vi "TriggeredHistogram10.vi"(7 "Last laser in":bool, 9 "Histogram in":u16[](array[numeric])=[0, 0, 0, 0, 0, 0, 0, 0, 0, 0], 10 "PMT 20bit in":bool[](array[boolean])=[FALSE, FALSE, FALSE, FALSE, FALSE, FALSE, FALSE, FALSE, FALSE, FALSE, FALSE, FALSE, FALSE, FALSE, FALSE, FALSE, FALSE, FALSE, FALSE, FALSE], 11 "Laser 10bit in":bool[](array[boolean])=[FALSE, FALSE, FALSE, FALSE, FALSE, FALSE, FALSE, FALSE, FALSE, FALSE]) -> (1 "Histogram out":u16[](array[numeric]))   [LabVIEW 2012]
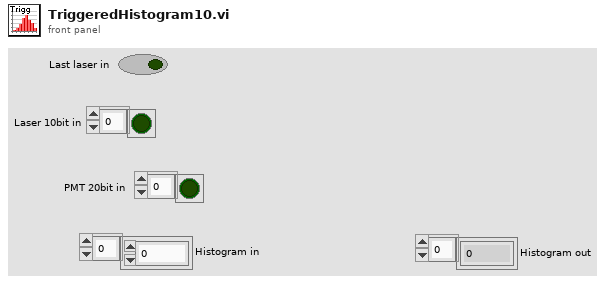
[diagram p1: front panel]
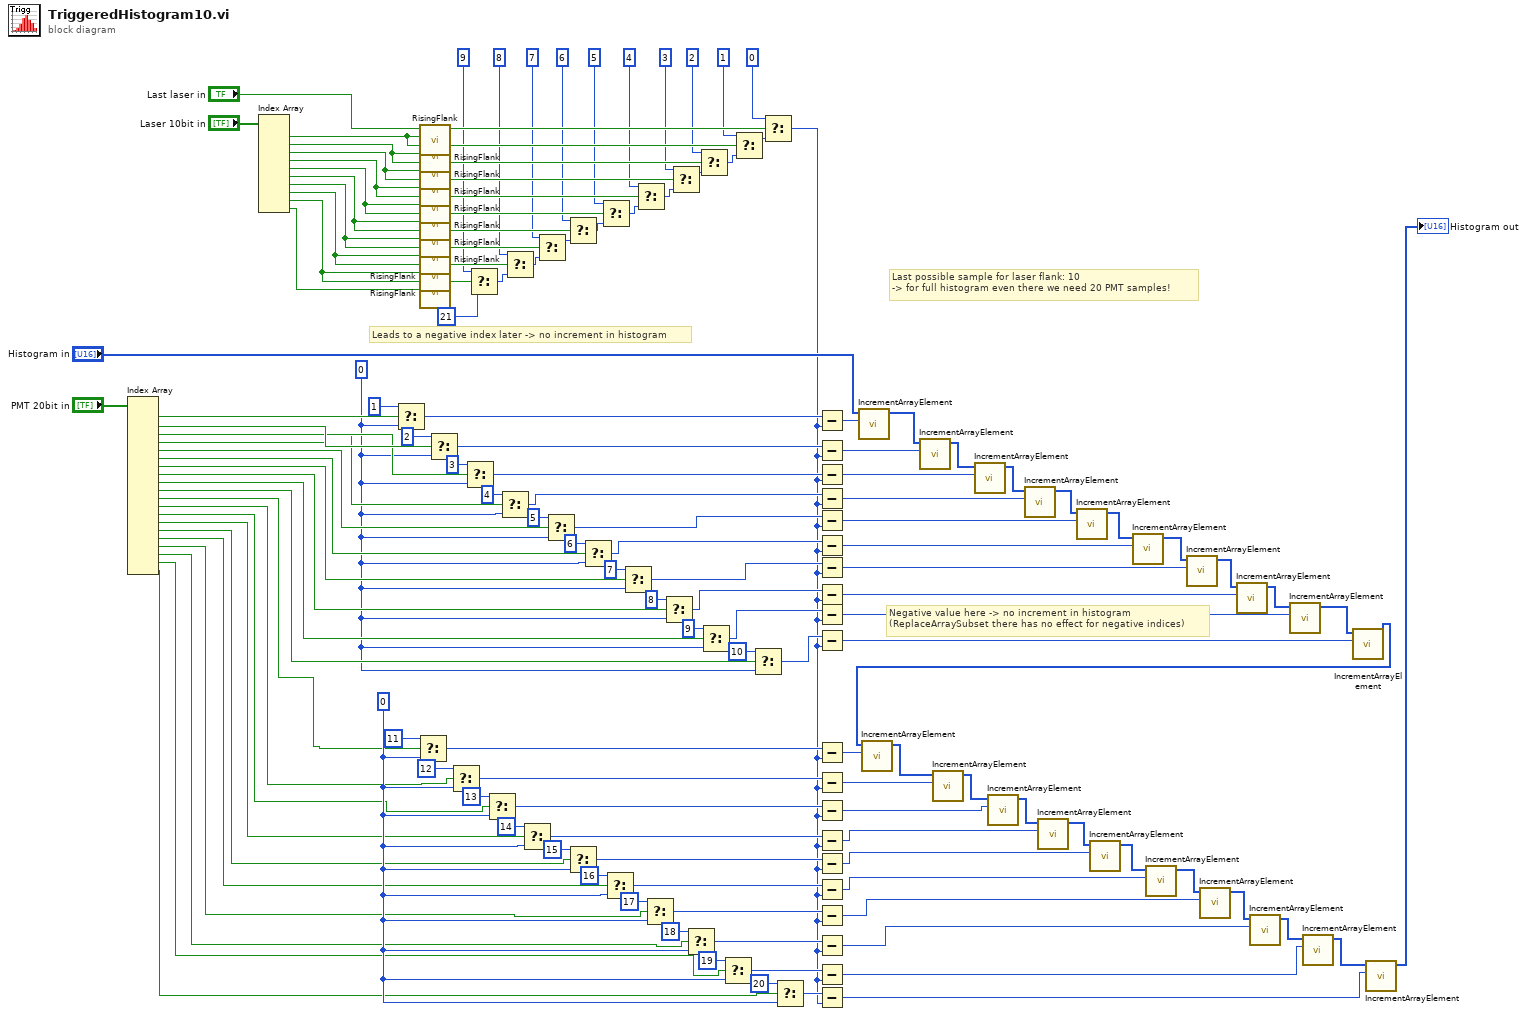
[diagram p0: block diagram]
diagram:
  w43 = 0 ("f")
  w84 = 0 ("f")
  # "Last possible sample for laser flank: 10\n-> for full histogram even there we need 20 PMT samples!"
  # "Leads to a negative index later -> no increment in histogram"
  # "Negative value here -> no increment in histogram\n(ReplaceArraySubset there has no effect for negative indices)"
  n1 = Index Array(array="PMT 20bit in") -> (element #1=w104:bool, element #2=w102:bool, element #3=w100:bool, element #4=w97:bool, element #5=w95:bool, element #6=w93:bool, element #7=w91:bool, element #8=w89:bool, element #9=w87:bool, element #10=w85:bool, element #11=w42:bool, element #12=w41:bool, element #13=w40:bool, element #14=w39:bool, element #15=w38:bool, element #16=w37:bool, element #17=w36:bool, element #18=w35:bool, element #19=w34:bool, element #20=w33:bool)  [unwired: 20 in]
  n2 = Index Array(array="Laser 10bit in") -> (element #1=w146:bool, element #2=w145:bool, element #3=w144:bool, element #4=w143:bool, element #5=w142:bool, element #6=w141:bool, element #7=w140:bool, element #8=w139:bool, element #9=w138:bool, element #10=w137:bool)  [unwired: 10 in]
  n3 = Select(t=1, s=w104, f=w84) -> (s? t:f=w83:i32)
  n4 = Select(t=11, s=w42, f=w43) -> (s? t:f=w32:i32)
  n5 = call "RisingFlank.vi"("2nd sample"=w146, "1st sample"="Last laser in") -> ("Rising flank?"=w136:bool)  [unwired: 7 in]
  n6 = call "RisingFlank.vi"("2nd sample"=w145, "1st sample"=w146) -> ("Rising flank?"=w133:bool)  [unwired: 7 in]
  n7 = call "RisingFlank.vi"("2nd sample"=w144, "1st sample"=w145) -> ("Rising flank?"=w132:bool)  [unwired: 7 in]
  n8 = call "RisingFlank.vi"("2nd sample"=w143, "1st sample"=w144) -> ("Rising flank?"=w131:bool)  [unwired: 7 in]
  n9 = call "RisingFlank.vi"("2nd sample"=w142, "1st sample"=w143) -> ("Rising flank?"=w130:bool)  [unwired: 7 in]
  n10 = call "RisingFlank.vi"("2nd sample"=w141, "1st sample"=w142) -> ("Rising flank?"=w129:bool)  [unwired: 7 in]
  n11 = call "RisingFlank.vi"("2nd sample"=w140, "1st sample"=w141) -> ("Rising flank?"=w128:bool)  [unwired: 7 in]
  n12 = call "RisingFlank.vi"("2nd sample"=w139, "1st sample"=w140) -> ("Rising flank?"=w127:bool)  [unwired: 7 in]
  n13 = call "RisingFlank.vi"("2nd sample"=w138, "1st sample"=w139) -> ("Rising flank?"=w126:bool)  [unwired: 7 in]
  n14 = call "RisingFlank.vi"("2nd sample"=w137, "1st sample"=w138) -> ("Rising flank?"=w125:bool)  [unwired: 7 in]
  n15 = Select(t=2, s=w102, f=w84) -> (s? t:f=w82:i32)
  n16 = Select(t=12, s=w41, f=w43) -> (s? t:f=w31:i32)
  n17 = Select(t=3, s=w100, f=w84) -> (s? t:f=w77:i32)
  n18 = Select(t=9 ("Insert index"), s=w125, f=21) -> (s? t:f=w109:i32)
  n19 = Select(t=13, s=w40, f=w43) -> (s? t:f=w30:i32)
  n20 = Select(t=4, s=w97, f=w84) -> (s? t:f=w76:i32)
  n21 = Select(t=8 ("Insert index"), s=w126, f=w109) -> (s? t:f=w111:i32)
  n22 = Select(t=14, s=w39, f=w43) -> (s? t:f=w29:i32)
  n23 = Select(t=7 ("Insert index"), s=w127, f=w111) -> (s? t:f=w113:i32)
  n24 = Select(t=5, s=w95, f=w84) -> (s? t:f=w75:i32)
  n25 = Select(t=6 ("Insert index"), s=w128, f=w113) -> (s? t:f=w115:i32)
  n26 = Select(t=15, s=w38, f=w43) -> (s? t:f=w28:i32)
  n27 = Select(t=6, s=w93, f=w84) -> (s? t:f=w74:i32)
  n28 = Select(t=5 ("Insert index"), s=w129, f=w115) -> (s? t:f=w117:i32)
  n29 = Select(t=16, s=w37, f=w43) -> (s? t:f=w27:i32)
  n30 = Select(t=7, s=w91, f=w84) -> (s? t:f=w73:i32)
  n31 = Select(t=4 ("Insert index"), s=w130, f=w117) -> (s? t:f=w119:i32)
  n32 = Select(t=17, s=w36, f=w43) -> (s? t:f=w26:i32)
  n33 = Select(t=8, s=w89, f=w84) -> (s? t:f=w72:i32)
  n34 = Select(t=3 ("Insert index"), s=w131, f=w119) -> (s? t:f=w122:i32)
  n35 = Select(t=18, s=w35, f=w43) -> (s? t:f=w25:i32)
  n36 = Select(t=2 ("Insert index"), s=w132, f=w122) -> (s? t:f=w124:i32)
  n37 = Select(t=9, s=w87, f=w84) -> (s? t:f=w71:i32)
  n38 = Select(t=19, s=w34, f=w43) -> (s? t:f=w24:i32)
  n39 = Select(t=1 ("Insert index"), s=w133, f=w124) -> (s? t:f=w134:i32)
  n40 = Select(t=10, s=w85, f=w84) -> (s? t:f=w70:i32)
  n41 = Select(t=0 ("Insert index"), s=w136, f=w134) -> (s? t:f=w22:i32)
  n42 = Select(t=20, s=w33, f=w43) -> (s? t:f=w23:i32)
  n43 = Subtract(x=w83, y=w22) -> (x-y=w80:i32)
  n44 = Subtract(x=w82, y=w22) -> (x-y=w78:i32)
  n45 = Subtract(x=w77, y=w22) -> (x-y=w69:i32)
  n46 = Subtract(x=w76, y=w22) -> (x-y=w66:i32)
  n47 = Subtract(x=w75, y=w22) -> (x-y=w65:i32)
  n48 = Subtract(x=w74, y=w22) -> (x-y=w62:i32)
  n49 = Subtract(x=w73, y=w22) -> (x-y=w60:i32)
  n50 = Subtract(x=w72, y=w22) -> (x-y=w59:i32)
  n51 = Subtract(x=w71, y=w22) -> (x-y=w58:i32)
  n52 = Subtract(x=w70, y=w22) -> (x-y=w57:i32)
  n53 = Subtract(x=w32, y=w22) -> (x-y=w20:i32)
  n54 = Subtract(x=w31, y=w22) -> (x-y=w10:i32)
  n55 = Subtract(x=w30, y=w22) -> (x-y=w9:i32)
  n56 = Subtract(x=w29, y=w22) -> (x-y=w8:i32)
  n57 = Subtract(x=w28, y=w22) -> (x-y=w7:i32)
  n58 = Subtract(x=w27, y=w22) -> (x-y=w6:i32)
  n59 = Subtract(x=w26, y=w22) -> (x-y=w5:i32)
  n60 = Subtract(x=w25, y=w22) -> (x-y=w4:i32)
  n61 = Subtract(x=w24, y=w22) -> (x-y=w3:i32)
  n62 = Subtract(x=w23, y=w22) -> (x-y=w2:i32)
  n63 = call "IncrementArrayElement.vi"("Index"=w80, "Histogram in"="Histogram in") -> ("Histogram out"=w79:u16[])  [unwired: 9 in]
  n64 = call "IncrementArrayElement.vi"("Index"=w78, "Histogram in"=w79) -> ("Histogram out"=w68:u16[])  [unwired: 9 in]
  n65 = call "IncrementArrayElement.vi"("Index"=w69, "Histogram in"=w68) -> ("Histogram out"=w67:u16[])  [unwired: 9 in]
  n66 = call "IncrementArrayElement.vi"("Index"=w66, "Histogram in"=w67) -> ("Histogram out"=w64:u16[])  [unwired: 9 in]
  n67 = call "IncrementArrayElement.vi"("Index"=w65, "Histogram in"=w64) -> ("Histogram out"=w63:u16[])  [unwired: 9 in]
  n68 = call "IncrementArrayElement.vi"("Index"=w62, "Histogram in"=w63) -> ("Histogram out"=w61:u16[])  [unwired: 9 in]
  n69 = call "IncrementArrayElement.vi"("Index"=w60, "Histogram in"=w61) -> ("Histogram out"=w56:u16[])  [unwired: 9 in]
  n70 = call "IncrementArrayElement.vi"("Index"=w59, "Histogram in"=w56) -> ("Histogram out"=w55:u16[])  [unwired: 9 in]
  n71 = call "IncrementArrayElement.vi"("Index"=w58, "Histogram in"=w55) -> ("Histogram out"=w54:u16[])  [unwired: 9 in]
  n72 = call "IncrementArrayElement.vi"("Index"=w57, "Histogram in"=w54) -> ("Histogram out"=w21:u16[])  [unwired: 9 in]
  n73 = call "IncrementArrayElement.vi"("Index"=w20, "Histogram in"=w21) -> ("Histogram out"=w13:u16[])  [unwired: 9 in]
  n74 = call "IncrementArrayElement.vi"("Index"=w10, "Histogram in"=w13) -> ("Histogram out"=w19:u16[])  [unwired: 9 in]
  n75 = call "IncrementArrayElement.vi"("Index"=w9, "Histogram in"=w19) -> ("Histogram out"=w18:u16[])  [unwired: 9 in]
  n76 = call "IncrementArrayElement.vi"("Index"=w8, "Histogram in"=w18) -> ("Histogram out"=w17:u16[])  [unwired: 9 in]
  n77 = call "IncrementArrayElement.vi"("Index"=w7, "Histogram in"=w17) -> ("Histogram out"=w16:u16[])  [unwired: 9 in]
  n78 = call "IncrementArrayElement.vi"("Index"=w6, "Histogram in"=w16) -> ("Histogram out"=w15:u16[])  [unwired: 9 in]
  n79 = call "IncrementArrayElement.vi"("Index"=w5, "Histogram in"=w15) -> ("Histogram out"=w14:u16[])  [unwired: 9 in]
  n80 = call "IncrementArrayElement.vi"("Index"=w4, "Histogram in"=w14) -> ("Histogram out"=w12:u16[])  [unwired: 9 in]
  n81 = call "IncrementArrayElement.vi"("Index"=w3, "Histogram in"=w12) -> ("Histogram out"=w11:u16[])  [unwired: 9 in]
  n82 = call "IncrementArrayElement.vi"("Index"=w2, "Histogram in"=w11) -> ("Histogram out"=→"Histogram out":u16[])  [unwired: 9 in]
